vi "Copy Graph to Clipboard.vi"(8 "error in (no error)":cluster{"状态":bool, "代码":i32, "源":string} caption="错误输入（无错误）", 11 "图形数据":T1={"UI引用"={"退出引用"=refnum, "保存引用"=refnum, "打开引用"=refnum, "导出引用"=refnum, "采集引用"=refnum, "配置引用"=refnum, "图形引用"=refnum, "清空引用"=refnum, "分析引用"=refnum, "状态引用"=refnum, "快照引用"=refnum}, "图形数据"={"数据"=[], "注释列表"=[], "游标列表"=[], "分析数据"=[]}, "用户定义"={"硬件配置"={"硬件引用句柄<替换此项>"="", "信号类型<替换该项>"=enum."Sine Wave"}, "分析配置"={"统计"=TRUE}, "新采集到数据时如何操作"=enum."Replace"}}) -> (0 "error out":cluster{"状态":bool, "代码":i32, "源":string} caption="错误输出")   [LabVIEW 2013]
doc: "将图形图像导出至剪贴板。"
uses:
  controls/Data.ctl
  controls/UI References.ctl
  controls/Graph Data.ctl
  <vilib>/Utility/miscctls.llb/LVAnnotationListTypeDef.ctl
  <vilib>/Utility/miscctls.llb/LVCursorListTypeDef.ctl
  controls/User Specified Data.ctl
  controls/HW Configuration.ctl
  controls/Simulated Signal Type.ctl
  controls/Analysis Configuration.ctl
  controls/New Data Behavior.ctl
panel:
  # "（向上滚动可查看大型数据簇）"
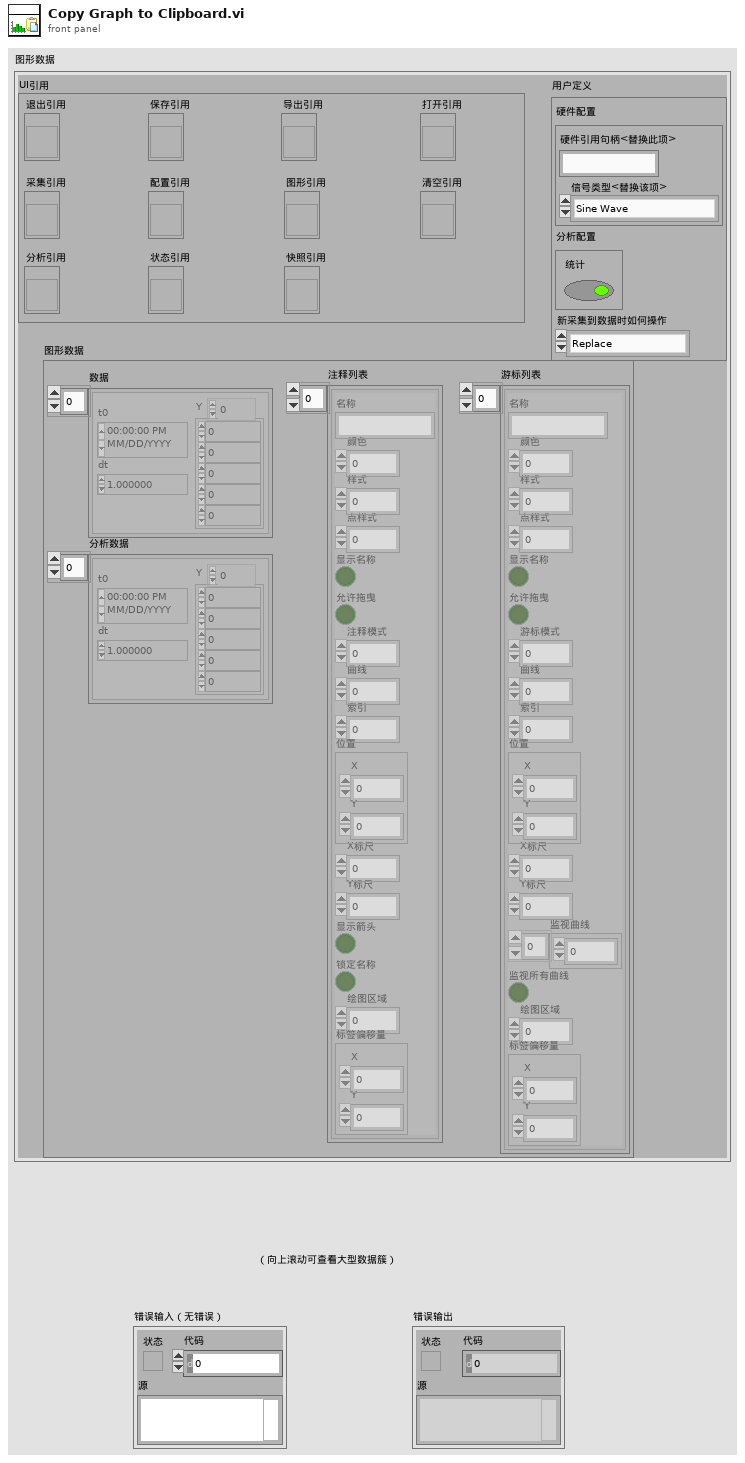
[diagram p1: front panel]
types:
  T1 = typedef "Data.ctl" = cluster{"UI引用":T2, "图形数据":T3, "用户定义":T6}
  T2 = typedef "UI References.ctl" = cluster{"退出引用":refnum<vi>, "保存引用":refnum<vi>, "打开引用":refnum<vi>, "导出引用":refnum<vi>, "采集引用":refnum<vi>, "配置引用":refnum<vi>, "图形引用":refnum<vi>, "清空引用":refnum<vi>, "分析引用":refnum<vi>, "状态引用":refnum<vi>, "快照引用":refnum<vi>}
  T3 = typedef "Graph Data.ctl" = cluster{"数据":waveform(dbl)[], "注释列表":T4, "游标列表":T5, "分析数据":waveform(dbl)[]}
  T4 = typedef "LVAnnotationListTypeDef.ctl" = cluster{"Name":string, "Color":u32, "Style":u8, "Point Style":u8, "Name Visible":bool, "Allow Drag":bool, "Annotation Mode":u32, "Plot":i32, "Index":i32, "Position":cluster{"X":dbl, "Y":dbl}, "X Scale":u32, "Y Scale":u32, "Show Arrow":bool, "Lock Name":bool, "Plot Area":i32, "Label Offset":cluster{"X":dbl, "Y":dbl}}[]
  T5 = typedef "LVCursorListTypeDef.ctl" = cluster{"Name":string, "Color":u32, "Style":u8, "Point Style":u8, "Name Visible":bool, "Allow Drag":bool, "Cursor Mode":u32, "Plot":i32, "Index":i32, "Position":cluster{"X":dbl, "Y":dbl}, "X Scale":u32, "Y Scale":u32, "Watch Plots":i32[], "Watch All Plots":bool, "Plot Area":i32, "Label Offset":cluster{"X":dbl, "Y":dbl}}[]
  T6 = typedef "User Specified Data.ctl" = cluster{"硬件配置":T7, "分析配置":T9, "新采集到数据时如何操作":T10}
  T7 = typedef "HW Configuration.ctl" = cluster{"硬件引用句柄<替换此项>":string, "信号类型<替换该项>":T8}
  T8 = typedef "Simulated Signal Type.ctl" = enum16{"Sine Wave", "Square Wave"}
  T9 = typedef "Analysis Configuration.ctl" = cluster{"统计":bool}
  T10 = typedef "New Data Behavior.ctl" = enum16{"Replace", "Overlay", "Append"}
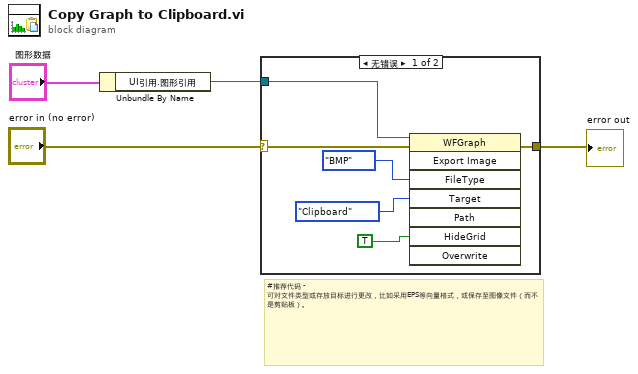
[diagram p0: block diagram]
diagram:
  # "#推荐代码 - 可对文件类型或存放目标进行更改，比如采用EPS等向量格式，或保存至图像文件（而不是剪贴板）。"
  n1 = Unbundle By Name("图形数据") -> ("UI引用.图形引用"=w3:refnum<vi>)
  n2 = case shown="无错误" "error in (no error)" {
    selector: "error in (no error)" -> [w5 w11]
    tunnel: w3 -> [w10 _]
    tunnel: [w6 w11] -> w2
    frame No Error {
      n3 = invoke class="WFGraph" method="Export Image"(reference=w10, error in=w5, "FileType"=enum32{"BMP", "EPS", "EMF", "PICT"}."BMP" ("File Type"), "Target"=enum32{"File", "Clipboard"}."Clipboard", "HideGrid"=TRUE ("Hide Grid")) -> (error out=w6:errorcluster)  [unwired: 3 in, 7 out]
    }
    frame Error {
    }
  }
  "error out" <- w2
